vi "writeToXML.vi"(8 "error in (no error)":errorcluster, 10 "ClassLabel":string, 11 "RADecTarget in":refnum<class "RADecTarget.lvclass">) -> (0 "error out":errorcluster, 2 "XMLout":string, 3 "RADecTarget out":refnum<class "RADecTarget.lvclass">)   [LabVIEW 2014, in "TCSDataDefinitions.lvlib" / "TCSCommand.lvlib" / "TargetConfiguration.lvlib" / "Target.lvlib" / "FixedTarget.lvlib" / "RADecTarget.lvclass"]
uses:
  RADecTarget.lvclass
  RADecTarget.lvclass/RADecTarget.ctl
  FixedTarget/FixedTarget.lvclass
  RADecParameters/RADecParameters.lvclass
  <userlib>/Common/XML/XMLGenerator/XMLGenerator.lvclass
  <userlib>/Common/XML/XMLAttributeGenerator/XMLAttributeGenerator.lvclass
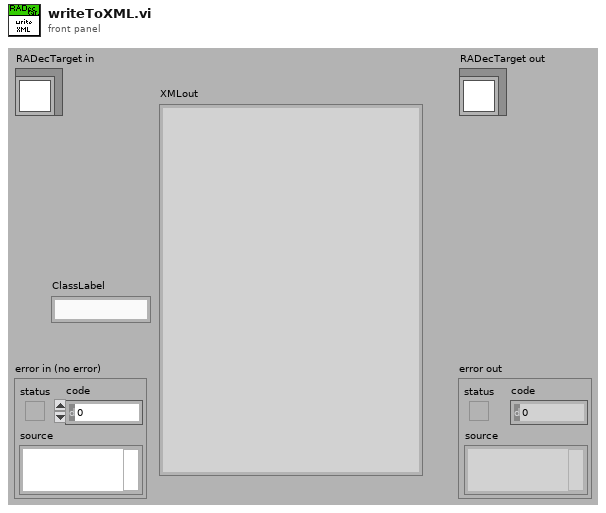
[diagram p1: front panel]
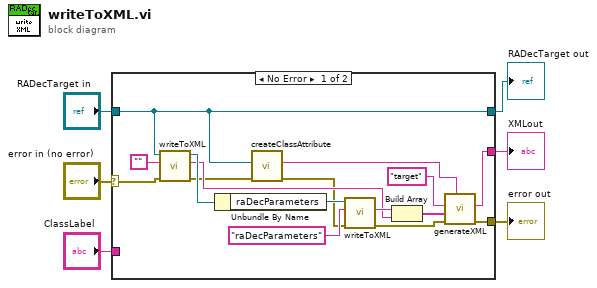
[diagram p0: block diagram]
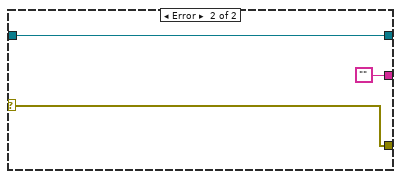
[diagram p2: hidden frame]
diagram:
  n1 = case shown="No Error" "error in (no error)" {
    selector: "error in (no error)" -> [w13 w25]
    tunnel: [w18 w25] -> w5
    tunnel: [w10 w24] -> w3
    tunnel: "RADecTarget in" -> [w10 w24]
    tunnel: [w17 ""] -> w2
    tunnel: "ClassLabel" -> [_ _]
    frame No Error {
      n2 = call-parent "writeToXML.vi"("error in (no error)"=w13, "ClassLabel"="", "FixedTarget in"=w10) -> ("error out"=w9:errorcluster, "XMLout"=w14:string, "FixedTarget out"=w16:refnum<class "RADecTarget.lvclass">)  [unwired: 6 in]
      n3 = Unbundle By Name(w16) -> ("raDecParameters"=w22:refnum<class "RADecParameters.lvclass">)
      n4 = call <userlib>:"createClassAttribute.vi"("error in (no error)"=w9, "LVClass In"=w10) -> ("error out"=w8:errorcluster, "AttributeString"=w7:string)  [unwired: 7 in, 1 out]
      n5 = call-dynamic "writeToXML.vi"("error in (no error)"=w8, "Class Label"="raDecParameters", "RADecParameters in"=w22) -> ("error out"=w11:errorcluster, "XML out"=w21:string)  [unwired: 6 in, 1 out]
      n6 = Build Array(w21, w14) -> (w20:string[])
      n7 = call <userlib>:"generateXML.vi"("attributeString"=w7, "error in"=w11, "childrenXML"=w20, "elementName"="target" ("Class Label")) -> ("error out"=w18:errorcluster, "XML out"=w17:string)  [unwired: 5 in, 1 out]
    }
    frame Error {
    }
  }
  "error out" <- w5
  "RADecTarget out" <- w3
  "XMLout" <- w2
